vi "GetParam.vi"(8 "error in (no error)":errorcluster caption="entrée d'erreur (pas d'erreur)", 11 "Precision_RFS.lvclass":refnum<class "Precision_RFS.lvclass">) -> (0 "error out":errorcluster caption="sortie d'erreur", 2 "precision_recall_fscore_support":T1={"beta"=1.0, "labels"=["None"], "pos_label"={"dtype_pos_label"="int", "pos_label"="1"}, "average"="None", "warn_for"=["precision", "recall", "f-score"], "sample_weight"=[], "zero_division"={"dtype_zero_division"="str", "zero_division"="warn"}, "Returns"="precision"}, 3 "Precision_RFS.lvclass":refnum<class "Precision_RFS.lvclass">)   [LabVIEW 2020, in "Precision_RFS.lvclass"]
doc: "Get Parameters"
uses:
  Precision_RFS.lvclass
  Precision_RFS.lvclass/Precision_RFS.ctl
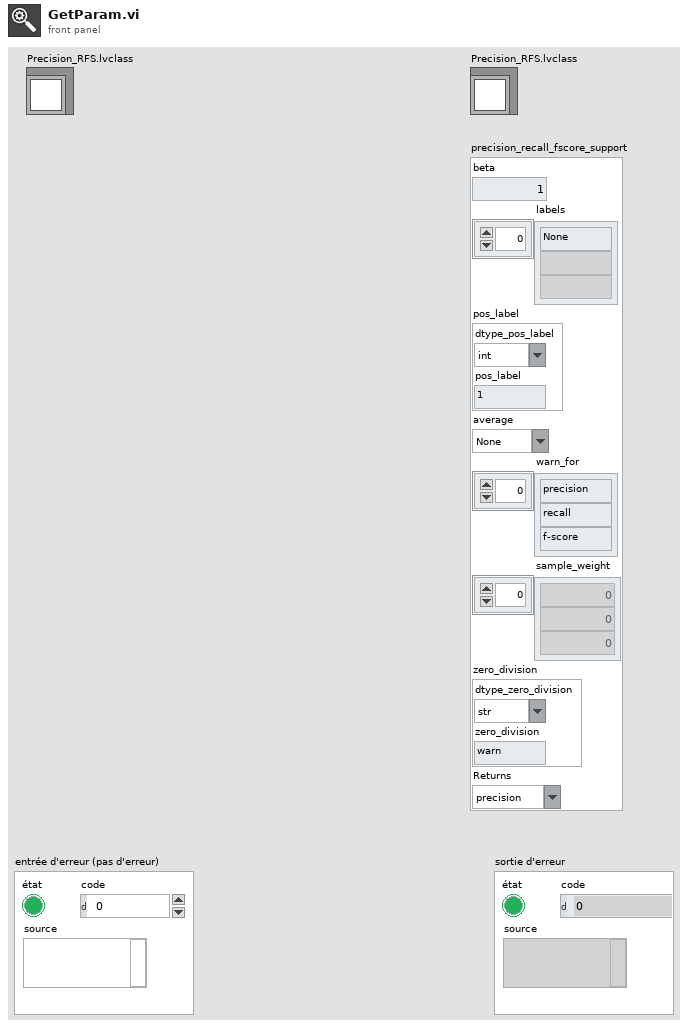
[diagram p1: front panel]
types:
  T1 = cluster{"beta":dbl, "labels":string[], "pos_label":cluster{"dtype_pos_label":string, "pos_label":string}, "average":string, "warn_for":string[], "sample_weight":dbl[], "zero_division":cluster{"dtype_zero_division":string, "zero_division":string}, "Returns":string}
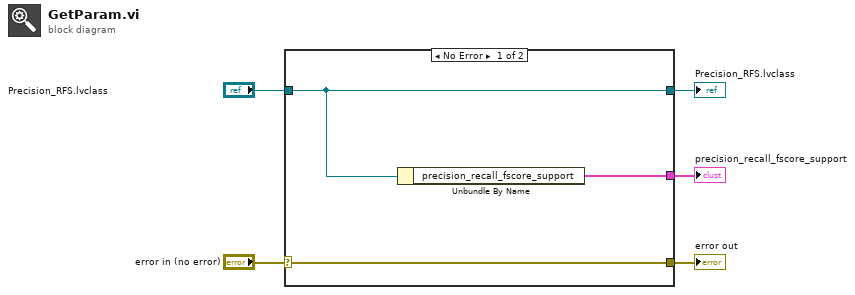
[diagram p0: block diagram]
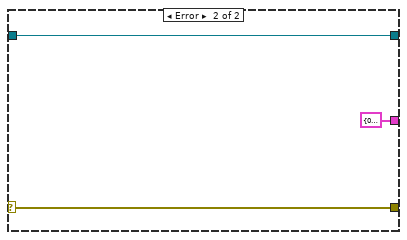
[diagram p2: hidden frame]
diagram:
  n1 = case shown="No Error" "error in (no error)" {
    selector: "error in (no error)" -> [w8 w10]
    tunnel: [w8 w10] -> w4
    tunnel: [w7 w11] -> w2
    tunnel: "Precision_RFS.lvclass" -> [w7 w11]
    tunnel: [w6 T1 {"beta"=0.0, "labels"=[], "pos_label"={"dtype_pos_label"="", "pos_label"=""}, "average"="", "warn_for"=[], "sample_weight"=[], "zero_division"={"dtype_zero_division"="", "zero_division"=""}, "Returns"=""} ("precision_recall_fscore_support")] -> w1
    frame No Error {
      n2 = Unbundle By Name(w7) -> ("precision_recall_fscore_support"=w6:T1)
    }
    frame Error {
    }
  }
  "error out" <- w4
  "Precision_RFS.lvclass" <- w2
  "precision_recall_fscore_support" <- w1
